vi "ZscanReadandConvert.vi"(0 "z/intensity memory address":u32) -> (1 "intensity profile":u16, 2 "z profile":u16, 3 "address out":u32)   [LabVIEW 2010]
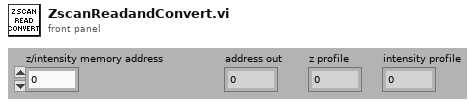
[diagram p1: front panel]
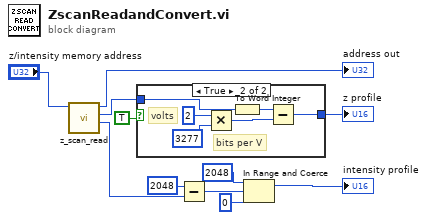
[diagram p0: block diagram]
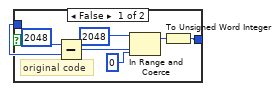
[diagram p2: hidden frame]
diagram:
  n1 = call "z_scan_read.vi"("address in"="z/intensity memory address") -> ("intensity"=w4:u16, "z-value"=w9:i16, "address out"=→"address out":u32)  [unwired: 8 in]
  n2 = case shown="True" TRUE {
    tunnel: w9 -> [w12 w24]
    tunnel: [w13 w23] -> w10
    frame False {
      # "original code"
      n3 = Subtract(x=i16 2048, y=w12) -> (x-y=w14:i16)
      n4 = In Range and Coerce(upper limit=i16 2048, x=w14, lower limit=i16 0) -> (coerced(x)=w15:i16)  [unwired: 1 out]
      n5 = To Unsigned Word Integer(number=w15) -> (unsigned 16bit integer=w13:u16)
    }
    frame True {
      # "bits per V"
      # "volts"
      n6 = Multiply(x=i16 2 ("y"), y=i16 3277) -> (x*y=w21:i16)
      n7 = To Word Integer(number=w24) -> (16bit integer=w19:i16)
      n8 = Subtract(x=w19, y=w21) -> (x-y=w23:i16)
    }
  }
  "z profile" <- w10
  n9 = Subtract(x=i16 2048, y=w4) -> (x-y=w8:u16)
  n10 = In Range and Coerce(upper limit=u16 2048, x=w8, lower limit=u16 0) -> (coerced(x)=→"intensity profile":u16)  [unwired: 1 out]
